vi "VPA QC General Section.vi"(10 "State Cluster":T1) -> (2 "State Cluster Out":T1)   [LabVIEW 2013]
uses:
  Controls/VPA QC State Data Cluster.ctl
  Controls/VPA QC General Cluster.ctl
  Controls/VPA QC State Enum.ctl
  Controls/VPA QC Bool Cluster.ctl
panel:
  in  "General Information Clust":T2
  in  "Help":bool
  in  "Cancel":bool
  in  "Save":bool
  # "Assembly Checklist"
  # "Assembly Checklist"
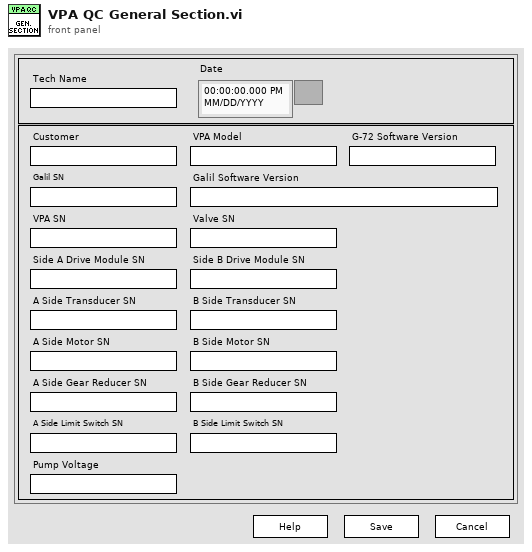
[diagram p1: front panel]
types:
  T1 = typedef "VPA QC State Data Cluster.ctl" = cluster{"XDCR 1":tag, "XDCR 2":tag, "General Information Clust":T2, "Assembly Checklist":cluster{"Ensure Drive Assembly checklist is completed.":bool, "Tighten Screws":bool, "Ensure VPA is wired correctly.":bool, "Ensure pump is running at voltage specified by customer.":bool}, "State":T3, "Manifold Leak Test Data":dbl[][], "Pressure Verification Test Data":dbl[][], "Flow Mode Verification Data":dbl[][], "DAQmx Error":errorcluster, "Bool Cluster":T4, "Leak Test Start Time":timestamp, "Pressure Test Start Time":timestamp, "Flow Test Start Time":timestamp, "Final Checklist cluster":cluster{"Check Fact Rest":bool, "Initialize Pump":bool, "Maintenance Hours":bool, "Clean Water Out":bool, "Covers":bool, "Screws":bool, "Wrap":bool, "Box":bool}, "Volts Constant":dbl, "Volume Constant A":dbl, "Volume Constant B":dbl, "Save File Path":path, "Comments Array":string[][]}
  T2 = typedef "VPA QC General Cluster.ctl" = cluster{"Tech Name":string, "Date":timestamp, "Customer":string, "VPA Model":string, "G-72 Software Version":string, "Galil SN":string, "Galil Software Version":string, "VPA SN":string, "Valve SN":string, "Side A Drive Module SN":string, "Side B Drive Module SN":string, "A Side Transducer SN":string, "B Side Transducer SN":string, "A Side Motor SN":string, "B Side Motor SN":string, "A Side Gear Reducer SN":string, "B Side Gear Reducer SN":string, "A Side Limit Switch SN":string, "B Side Limit Switch SN":string, "Pump Voltage":string}
  T3 = typedef "VPA QC State Enum.ctl" = enum16{"General Information", "XDCR and LS Check", "Check Pump Function", "Manifold/Cylinder Leak Test", "Exit"}
  T4 = typedef "VPA QC Bool Cluster.ctl" = cluster{"Assembly":bool, "Gen":bool, "XDCR and LS Setup":bool, "Verify Pump Operation":bool, "Leak Test":bool, "Calibrate XDCRs":bool, "P Mode Verify":bool, "F Mode Verify":bool, "Vol Calibration":bool, "Final Checklist":bool}
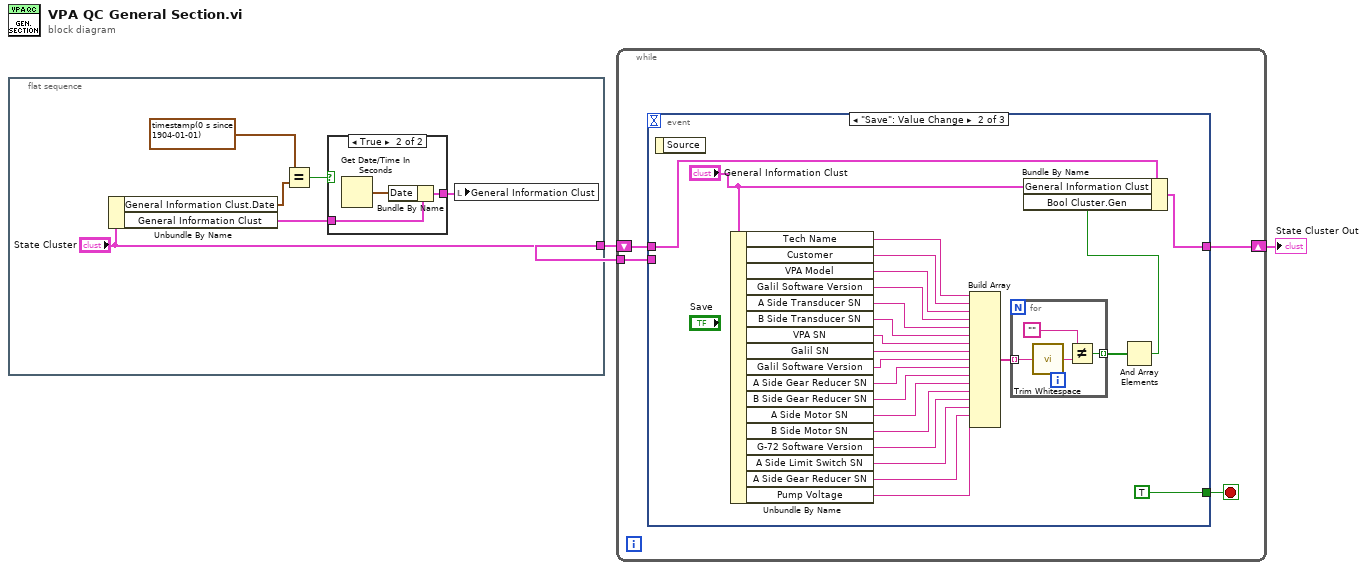
[diagram p0: block diagram]
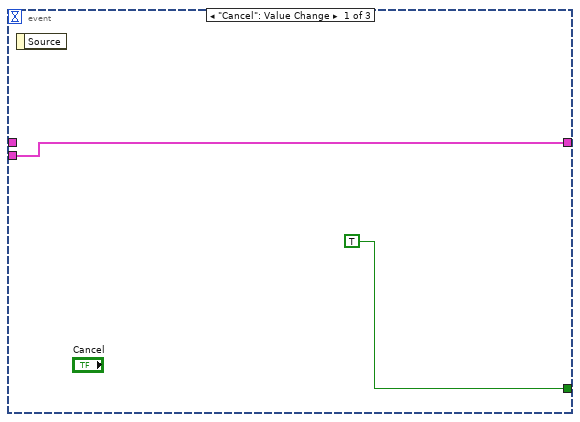
[diagram p3: hidden frame]
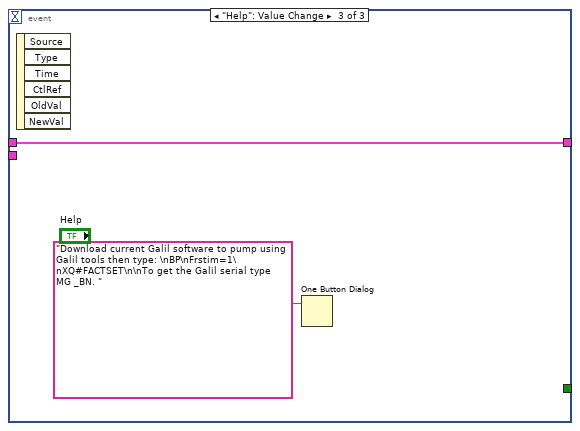
[diagram p4: hidden frame]
diagram:
  n1 = flat-sequence {
    tunnel: ["State Cluster"] -> w2
    frame #0 {
      n2 = Unbundle By Name("State Cluster") -> ("General Information Clust.Date"=w5:timestamp, "General Information Clust"=w7:T2)
      n3 = Equal?(x=timestamp(0 s since 1904-01-01) ("General Information Clust.Date"), y=w5) -> (x = y?=w3:bool)
      n4 = case shown="True" w3 {
        tunnel: w7 -> [w9 w12]
        tunnel: [w9 w10] -> w6
        frame False {
        }
        frame True {
          n5 = Get Date/Time In Seconds() -> (seconds since 1Jan1904=w11:timestamp)
          n6 = Bundle By Name(cluster=w12, "Date"=w11) -> (w10:T2)
        }
      }
      n7 = local write "General Information Clust"(w6) -> ()
    }
  }
  n8 = while {
    shift-right: [w14] -> w1
    shift-left: w2 -> [w15]
    tunnel: w2 -> [w13]
    stop <- w16 stop-if-true
    n9 = event shown="[1] \"Save\": Value Change" {
      selector: _ -> [_ _ _]
      dyn-events: _ -> [_ _ _]
      timeout: _ -> [_ _ _]
      tunnel: [TRUE TRUE _] -> w16
      tunnel: w15 -> [_ w41 w48]
      tunnel: [w17 w40 w48] -> w14
      tunnel: w13 -> [w17 _ _]
      event "Cancel": Value Change {
        n10 = event-data() -> ()  [unwired: 1 in, 1 out]
      }
      event "Save": Value Change {
        n11 = event-data() -> ()  [unwired: 1 in, 1 out]
        n12 = Unbundle By Name("General Information Clust") -> ("Tech Name"=w38:string, "Customer"=w37:string, "VPA Model"=w36:string, "Galil Software Version"=w35:string, "A Side Transducer SN"=w34:string, "B Side Transducer SN"=w33:string, "VPA SN"=w32:string, "Galil SN"=w31:string, "Galil Software Version"=w30:string, "A Side Gear Reducer SN"=w29:string, "B Side Gear Reducer SN"=w28:string, "A Side Motor SN"=w27:string, "B Side Motor SN"=w26:string, "G-72 Software Version"=w25:string, "A Side Limit Switch SN"=w24:string, "A Side Gear Reducer SN"=w23:string, "Pump Voltage"=w22:string)
        n13 = Build Array(w38, w37, w36, w35, w34, w33, w32, w31, w30, w29, w28, w27, w26, w25, w24, w23, w22) -> (w21:string[])
        n14 = for {
          tunnel: w21 -> [w44] mode=indexing
          tunnel: [w45] -> w20 mode=indexing
          n15 = call <vilib>:"Trim Whitespace.vi"("string"=w44) -> ("trimmed string"=w43:string)  [unwired: 1 in]
          n16 = Not Equal?(x="", y=w43) -> (x != y?=w45:bool)
        }
        n17 = And Array Elements(Boolean array=w20) -> (logical AND=w19:bool)
        n18 = Bundle By Name(cluster=w41, "General Information Clust"="General Information Clust", "Bool Cluster.Gen"=w19) -> (w40:T1)
      }
      event "Help": Value Change {
        n19 = event-data() -> ()  [unwired: 1 in, 6 out]
        n20 = One Button Dialog(message="Download current Galil software to pump using  Galil tools then type: \nBP\nFrstim=1\nXQ#FACTSET\n\nTo get the Galil serial type MG _BN. ") -> ()  [unwired: 1 in, 1 out]
      }
    }
  }
  "State Cluster Out" <- w1
